vi "linkam.setRate.vi"(8 "error in (no error)":errorcluster, 10 "rate":dbl format="%.2g", 11 "VISA resource name in":refnum<visa-resource-name>) -> (0 "error out":errorcluster, 3 "VISA resource name out":refnum<visa-resource-name>)   [LabVIEW 8.6]
panel:
  in  "Serial Settings:Number of Bytes at Serial Port":u32
  out "concatenated string":string
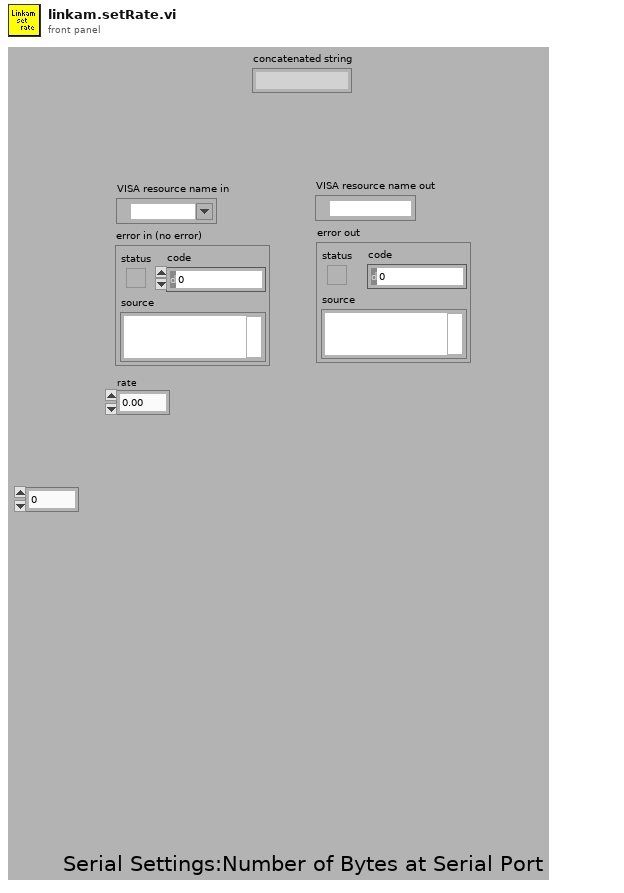
[diagram p1: front panel]
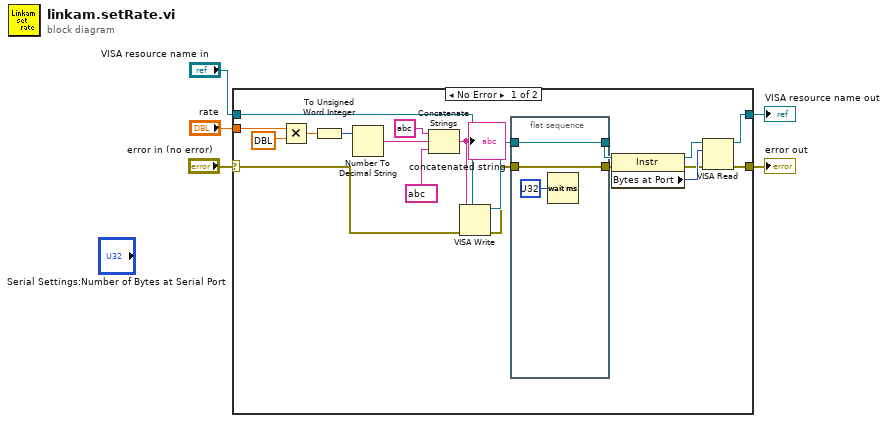
[diagram p0: block diagram]
diagram:
  n1 = case shown="No Error" "error in (no error)" {
    selector: "error in (no error)" -> [w23 w29]
    tunnel: [w21 w29] -> w3
    tunnel: [w22 w28] -> w2
    tunnel: "VISA resource name in" -> [w24 w28]
    tunnel: "rate" -> [w15 _]
    frame #0 {
      n2 = Multiply(x=w15, y=dbl ?) -> (x*y=w14:dbl)
      n3 = To Unsigned Word Integer(number=w14) -> (unsigned 16bit integer=w18:u16)
      n4 = Number To Decimal String(number=w18) -> (decimal integer string=w19:string)  [unwired: 1 in]
      n5 = Concatenate Strings(string ?, w19, string ? ("string")) -> (w17:string)
      "concatenated string" <- w17
      n6 = VISA Write(VISA resource name=w24, write buffer=w17, error in (no error)=w23) -> (VISA resource name out=w11:refnum<visa-resource-name>, error out=w9:errorcluster)  [unwired: 1 out]
      n7 = flat-sequence {
        tunnel: w11 -> [w27]
        tunnel: [w27] -> w10
        tunnel: w9 -> [w26]
        tunnel: [w26] -> w8
        frame #0 {
          n8 = Wait (ms)(milliseconds to wait=u32 ?) -> ()  [unwired: 1 out]
        }
      }
      n9 = property class="Instr"(reference=w10, error in=w8) -> (reference out=w6:refnum<visa-resource-name>, error out=w7:errorcluster, "Bytes at Port"=w12:u32)
      n10 = VISA Read(VISA resource name=w6, byte count=w12, error in (no error)=w7) -> (VISA resource name out=w22:refnum<visa-resource-name>, error out=w21:errorcluster)  [unwired: 2 out]
    }
    frame #1 {
    }
  }
  "VISA resource name out" <- w2
  "error out" <- w3
